vi "dll_freeBox.vi"(8 "error in (no error)":errorcluster, 11 "p_box":i32) -> (0 "error out":errorcluster)   [LabVIEW 2020, in "box.lvlib"]
uses:
  box.lvlib
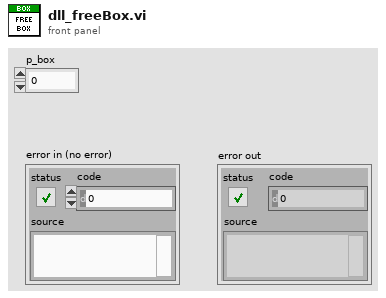
[diagram p1: front panel]
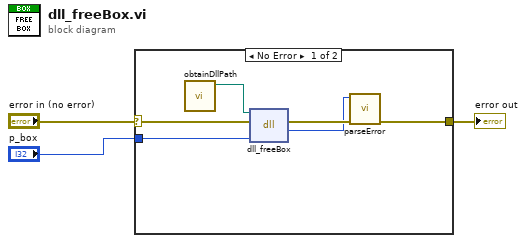
[diagram p0: block diagram]
diagram:
  n1 = case shown="No Error" "error in (no error)" {
    selector: "error in (no error)" -> [w9 w10]
    tunnel: "p_box" -> [w8 _]
    tunnel: [w6 w10] -> w1
    frame No Error {
      n2 = call "obtainDllPath.vi"() -> ("box.dll path"=w4:path)  [unwired: 11 in]
      n3 = dll-call lib="box.dll" fn="dll_freeBox"(path in=w4, error in=w9, "p_box"=w8) -> (error out=w7:errorcluster, "return type"=w5:i32)  [unwired: 2 in, 1 out]
      n4 = call "parseError.vi"("error in (no error)"=w7, "status code"=w5) -> ("error out"=w6:errorcluster)  [unwired: 9 in]
    }
    frame Error {
    }
  }
  "error out" <- w1
